vi "Load Category.vi"(8 "error in (no error)":errorcluster, 10 "Category Base Path":path, 11 "Home in":refnum<class "Home.lvclass">) -> (0 "error out":errorcluster, 3 "Home out":refnum<class "Home.lvclass">)   [LabVIEW 2015, in "Category Library.lvlib" / "Home.lvclass"]
uses:
  Home.lvclass
  <vilib>/picture/picture.llb/imagedata.ctl
  Category/Category.lvclass/Category.ctl
  Category/Write Icon Raw.vi
  Category/Write Name.vi
  Category/Write Weight.vi
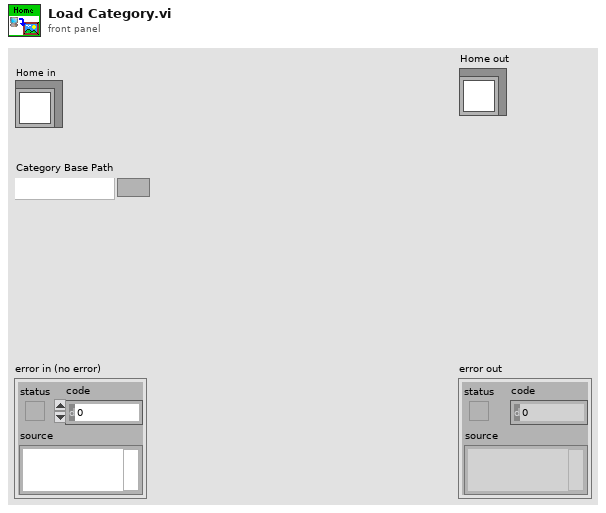
[diagram p1: front panel]
types:
  T1 = typedef "imagedata.ctl" = cluster{"image type":i32, "image depth":i32, "image":u8[], "mask":u8[], "colors":u32[], "Rectangle":cluster{"left":i16, "top":i16, "right":i16, "bottom":i16}}
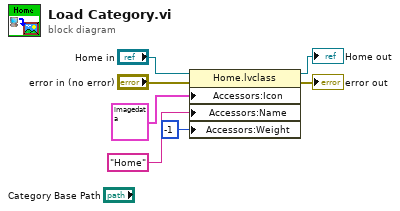
[diagram p0: block diagram]
diagram:
  n1 = property class="Home.lvclass"(reference="Home in", error in="error in (no error)", "Accessors:Icon"=T1 {"image type"=0, "image depth"=32, "image"=array[16384 elements], "mask"=[0, 0, 0, 0, 0, 0, 0, 0, 0, 0, 0, 0, 0, 0, 0, 0, 0, 0, 0, 0, 0, 0, 0, 0, 0, 0, 0, 0, 0, 0, 0, 0, 0, 0, 0, 0, 0, 0, 0, 0, 0, 0, 0, 0, 0, 0, 0, 0, 0, 0, 0, 0, 0, 0, 0, 0, 0, 0, 0, 0, 0, 0, 0, 0, 0, 0, 0, 0, 0, 0, 0, 0, 0, 0, 0, 0, 0, 0, 0, 0, 0, 0, 0, 3, 192, 0, 0, 0, 0, 0, 0, 15, 240, 0, 0, 0, 0, 0, 0, 63, 252, 63, 0, 0, 0, 0, 0, 127, 254, 63, 128, 0, 0, 0, 1, 255, 255, 191, 128, 0, 0, 0, 7, 255, 255, 255, 128, 0, 0, 0, 31, 255, 255, 255, 128, 0, 0, 0, 127, 255, 255, 255, 128, 0, 0, 0, 255, 255, 255, 255, 128, 0, 0, 3, 255, 255, 255, 255, 192, 0, 0, 15, 255, 255, 255, 255, 240, 0, 0, 63, 255, 255, 255, 255, 252, 0, 0, 127, 255, 255, 255, 255, 254, 0, 1, 255, 255, 255, 255, 255, 255, 128, 3, 255, 255, 255, 255, 255, 255, 192, 3, 255, 255, 255, 255, 255, 255, 192, 3, 255, 255, 255, 255, 255, 255, 192, 1, 255, 255, 255, 255, 255, 255, 128, 1, 247, 255, 255, 255, 255, 239, 128, 0, 199, 255, 255, 255, 255, 227, 0, 0, 7, 255, 255, 255, 255, 224, 0, 0, 7, 255, 255, 255, 255, 224, 0, 0, 7, 255, 255, 255, 255, 224, 0, 0, 7, 255, 255, 255, 255, 224, 0, 0, 7, 255, 255, 255, 255, 224, 0, 0, 7, 255, 255, 255, 255, 224, 0, 0, 7, 255, 255, 255, 255, 224, 0, 0, 7, 255, 255, 255, 255, 224, 0, 0, 7, 255, 255, 255, 255, 224, 0, 0, 7, 255, 255, 255, 255, 224, 0, 0, 7, 255, 255, 255, 255, 224, 0, 0, 7, 255, 224, 7, 255, 224, 0, 0, 7, 255, 224, 7, 255, 224, 0, 0, 7, 255, 224, 7, 255, 224, 0, 0, 7, 255, 224, 7, 255, 224, 0, 0, 7, 255, 224, 7, 255, 224, 0, 0, 7, 255, 224, 7, 255, 224, 0, 0, 7, 255, 224, 7, 255, 224, 0, 0, 7, 255, 224, 7, 255, 224, 0, 0, 7, 255, 224, 7, 255, 224, 0, 0, 7, 255, 224, 7, 255, 224, 0, 0, 7, 255, 224, 7, 255, 224, 0, 0, 7, 255, 224, 7, 255, 224, 0, 0, 7, 255, 224, 7, 255, 224, 0, 0, 0, 0, 0, 0, 0, 0, 0, 0, 0, 0, 0, 0, 0, 0, 0, 0, 0, 0, 0, 0, 0, 0, 0, 0, 0, 0, 0, 0, 0, 0, 0, 0, 0, 0, 0, 0, 0, 0, 0, 0, 0, 0, 0, 0, 0, 0, 0, 0, 0, 0, 0, 0, 0, 0, 0, 0, 0, 0, 0, 0, 0, 0, 0, 0, 0, 0, 0, 0, 0, 0, 0, 0, 0, 0, 0, 0, 0, 0, 0], "colors"=[], "Rectangle"={"left"=0, "top"=0, "right"=64, "bottom"=64}} ("image data"), "Accessors:Name"="Home" ("Name"), "Accessors:Weight"=-1 ("Weight")) -> (reference out=→"Home out":refnum<class "Home.lvclass">, error out=→"error out":errorcluster)
